vi "Check Stale Clients.vi"(8 "error in (no error)":errorcluster, 11 "Messaging Server Module in":refnum<class "Messaging Server Module.lvclass">) -> (0 "error out":errorcluster, 3 "Messaging Server Module out":refnum<class "Messaging Server Module.lvclass">)   [LabVIEW 2020, in "Volatus.lvlib" / "Messaging Server Module.lvclass"]
uses:
  Messaging Server Module.lvclass
  Messaging Server Module.lvclass/Messaging Server Module.ctl
  MessageQ/MessageQ.lvclass
  Msg Client State.ctl
  Volatus.lvlib
  Module/Module.lvclass
  VolatusAPI/VolatusAPI.lvclass
  Event Level.ctl
  C:/dev/lv20CE/relink/lv-volatus/Volatus/Module/Module.lvclass
  C:/dev/lv20CE/relink/lv-volatus/Volatus/Messaging Server Module/Messaging Server Module.lvclass
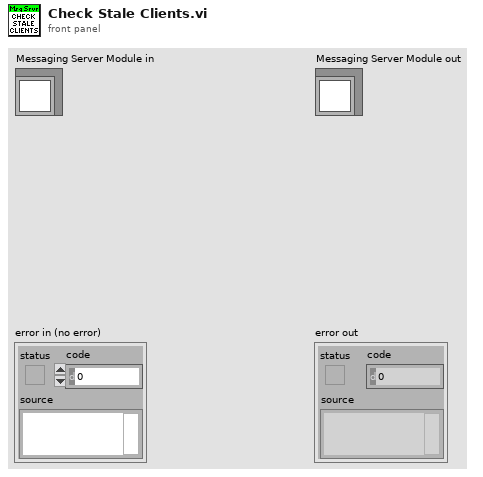
[diagram p1: front panel]
types:
  T1 = typedef "Volatus.lvlib/Msg Client State.ctl" = enum16{"Unknown", "Handshake", "Connected", "Closing"}
  T2 = typedef "Volatus.lvlib/Event Level.ctl" = enum16{"Debug", "Info", "Warning", "Error"}
  T3 = typedef "Volatus.lvlib/Messaging Server Module.lvclass/Client Info.ctl" = cluster{"MsgQ":refnum<class "MessageQ.lvclass">, "Address":string, "Port":u16, "Client State":T1, "Last Update":dbl, "Node":string, "Alias":string}
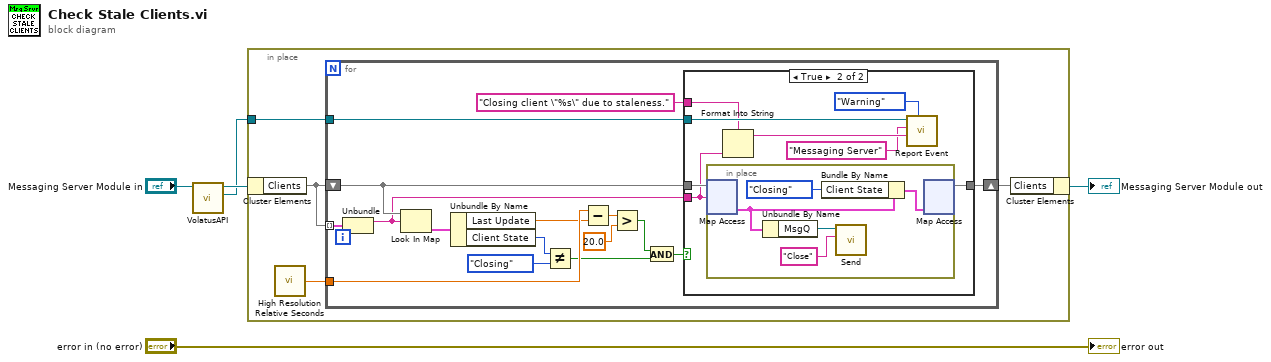
[diagram p0: block diagram]
diagram:
  n1 = call "VolatusAPI.vi"("Module in"="Messaging Server Module in") -> ("VolatusAPI"=w1:refnum<class "VolatusAPI.lvclass">, "Module out"=w2:refnum<class "Messaging Server Module.lvclass">)  [unwired: 9 in]
  n2 = in-place {
    in-place-border: w1 -> [w6]
    n3 = in-place-cluster #1(w2) -> ("Clients"=w9:map{string, T3})
    n4 = call <vilib>:"High Resolution Relative Seconds.vi"() -> ("relative seconds"=w8:dbl)
    n5 = for {
      shift-right: [w17] -> w7
      shift-left: w9 -> [w19]
      tunnel: w9 -> [w25] mode=indexing
      tunnel: w8 -> [w23]
      tunnel: w6 -> [w11]
      n6 = Unbundle(w25) -> ("Endpoint"=w18:string)  [unwired: 1 out]
      n7 = Look In Map(map=w19, key=w18) -> (value=w24:T3)  [unwired: 1 in, 1 out]
      n8 = Unbundle By Name(w24) -> ("Last Update"=w22:dbl, "Client State"=w16:T1)
      n9 = Not Equal?(x=w16, y=Msg_Client_State."Closing") -> (x != y?=w14:bool)
      n10 = Subtract(x=w23, y=w22) -> (x-y=w21:dbl)
      n11 = Greater?(x=w21, y=20.0) -> (0:w13:bool)
      n12 = And(x=w13, y=w14) -> (x .and. y?=w12:bool)
      n13 = case shown="True" w12 {
        tunnel: w19 -> [w26 w34]
        tunnel: w18 -> [_ w29]
        tunnel: [w26 w33] -> w17
        tunnel: w11 -> [_ w32]
        tunnel: "Closing client \"%s\" due to staleness." -> [_ w30]
        frame False {
        }
        frame True {
          n14 = in-place {
            n15 = in-place-map #2(w34, w29) -> (w37:T3)  [unwired: 1 in, 1 out]
            n16 = Unbundle By Name(w37) -> ("MsgQ"=w39:refnum<class "MessageQ.lvclass">)
            n17 = Bundle By Name(cluster=w37, "Client State"=Msg_Client_State."Closing") -> (w35:T3)
            n18 = call "Send.vi"("ID"="Close", "MessageQ in"=w39) -> ()  [unwired: 8 in, 2 out]
            n19 = in-place-map #2(w35) -> (w33:map{string, T3})  [unwired: 1 in, 2 out]
          }
          n20 = Format Into String(format string=w30, w29) -> (resulting string=w28:string)  [unwired: 2 in, 1 out]
          n21 = call "Report Event.vi"("Level (Info)"=Event_Level."Warning", "Message"=w28, "Context"="Messaging Server", "VolatusAPI in"=w32) -> ()  [unwired: 6 in, 2 out]
        }
      }
    }
    n22 = in-place-cluster #1("Clients"=w7) -> (→"Messaging Server Module out":refnum<class "Messaging Server Module.lvclass">)
  }
  "error out" <- "error in (no error)"
